vi "R_out.vi"(1 "install path":path=path "C:/Program Files (x86)/National Instruments/LabLinda", 5 "IN VARIANT":variant, 7 "Ip":string, 9 "Name in":string, 11 "error in (no error)":errorcluster) -> (10 "Operation Ok":bool, 15 "error out":errorcluster)   [LabVIEW 2015]
doc: "REMOTE OUT"
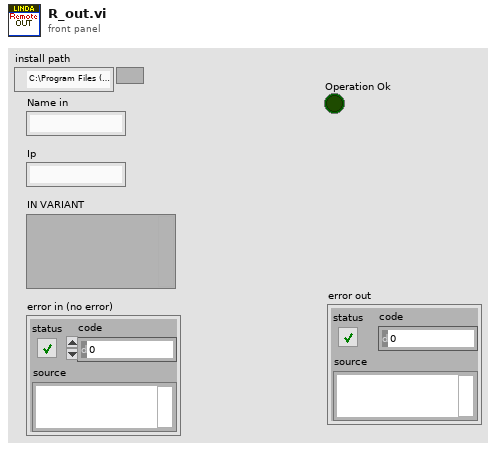
[diagram p1: front panel]
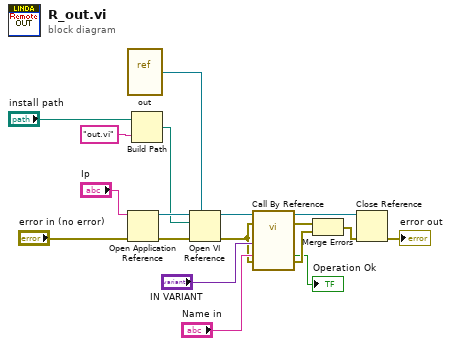
[diagram p0: block diagram]
diagram:
  n1 = vi-ref "out.vi"() -> (w12:refnum<vi>)
  n2 = Open Application Reference(8:"error in (no error)", 11:"Ip") -> (0:w13:errorcluster, 3:w16:refnum<vi>)  [unwired: 2 in]
  n3 = Build Path(base path="install path", name or relative path="out.vi") -> (appended path=w14:path)
  n4 = Open VI Reference(type specifier VI Refnum (for type only)=w12, application reference (local)=w16, vi path=w14, error in (no error)=w13) -> (vi reference=w11:refnum<vi>, error out=w4:errorcluster)  [unwired: 2 in]
  n5 = call-by-ref "?"(reference=w11, error in=w4, "IN VARIANT"="IN VARIANT", "Name in"="Name in", 11:"error in (no error)"=w4) -> (reference out=w7:refnum<vi>, error out=w10:errorcluster, "Operation Ok"=→"Operation Ok":bool, 15:"error out"=w9:errorcluster)  [unwired: 11 in]
  n6 = Merge Errors(w10, w9) -> (w8:errorcluster)
  n7 = Close Reference(reference=w7, error in (no error)=w8) -> (error out=→"error out":errorcluster)
